vi "Process.vi"(0 "WaveformAddressSpace in":refnum<class "WaveformAddressSpace.lvclass">, 5 "Data":sgl[](array[numeric])=[0.0, 0.0, 0.0, 0.0], 9 "Iteration":i32, 11 "error in (no error)":errorcluster, 12 "FirstIteration":bool) -> (4 "WaveformAddressSpace out":refnum<class "WaveformAddressSpace.lvclass">, 6 "Acq Loop Ticks":u32, 10 "stop":bool, 15 "error out":errorcluster)   [LabVIEW 2017, in "WaveformAddressSpace.lvclass"]
uses:
  WaveformAddressSpace.lvclass
  WaveformAddressSpace.lvclass/WaveformAddressSpace.ctl
  <vilib>/rvi/DataTransferAndStorage/Container/Common/niFpgaContainerExecOnDevCompGetState.vi
  <vilib>/rvi/Emulation/niFpgaEmulationIsFPGAContextNoSignature.vi
  <vilib>/rvi/DataTransferAndStorage/Container/Common/niFpgaContainerGetUniqueNameForEmu.vi
  <vilib>/rvi/Memory/Memory_Emulation/niFpgaMemoryEmulationCacheClearOnFirstRun.vi
  <vilib>/rvi/Memory/Memory_Emulation/nirvimemoryEmulationManagerCache_MakeExclusive.vi
  <vilib>/rvi/Memory/Memory_Emulation/niFpgaMemoryEmulationValidateCache.vi
  <vilib>/rvi/Memory/Memory_Emulation/nirvimemoryEmulationManagerCache_InsertValue.vi
  <vilib>/Utility/error.llb/Clear Errors.vi
  <vilib>/rvi/Memory/Memory_Emulation/nirvimemoryEmulationManagerCache_ReleaseExclusive.vi
  <vilib>/rvi/Memory/Memory_Emulation/nirvimemoryEmulationManagerCache_GetValue.vi
  <vilib>/rvi/Memory/Memory_Emulation/nirvimemoryEmulationManagerCache_SetValue.vi
  <vilib>/rvi/Emulation/niFpgaProcessEmulError.vi
  <vilib>/rvi/Emulation/niFpgaSctlEmulationGetInTimedLoop.vi
  <vilib>/rvi/errors/niFpgaSetErrorForExecOnDevCompSimple.vi
  <vilib>/rvi/eio/common/nirviEmuReportErrorAndStop.vi
  <vilib>/rvi/FIFO/Fifo_Resource/nirvififoEmulationSetSize.vi
  <vilib>/rvi/FIFO/Fifo_Resource/nirviFifoEmulationQueueMgr.vi
  <instcachedir>/0/nirviFifoEmulationQueueMgr_E5CAEC123FF24DC58D834DCA3CDAA9B5.lvgen/nirviFifoEmulationQueueMgr_E5CAEC123FF24DC58D834DCA3CDAA9B5_002.vi
  <vilib>/rvi/FIFO/Fifo_Resource/nirvififoEmulationDetermineInputValidOut.vi
  <vilib>/rvi/FIFO/Fifo_Resource/nirvififoEmulationCreateLock.vi
  <vilib>/rvi/FIFO/Fifo_Resource/nirvififoEmulationObtainLock.vi
  <vilib>/rvi/FIFO/Fifo_Resource/nirvififoEmulationReleaseLock.vi
  <vilib>/rvi/occurrence/nirviWaitOnOccurrenceBase.vi
  <vilib>/rvi/errors/nirviReportUnexpectedCaseInternalError.vi
  <vilib>/rvi/errors/nirviReportUnexpectedCaseInternalError (U32).vi
  <vilib>/rvi/interface/RandomDataEmulation/niFpgaRandomDataHandleErrors.vi
  <vilib>/rvi/DataTransferAndStorage/Container/XNode/niFpgaContainer.xnode
  <vilib>/rvi/DataTransferAndStorage/Register/Emulation/niFpgaRegisterEmulationRefIn.vi
  <vilib>/rvi/FIFO/Fifo_Resource/niFpgaFifoEmulationRefIn.vi
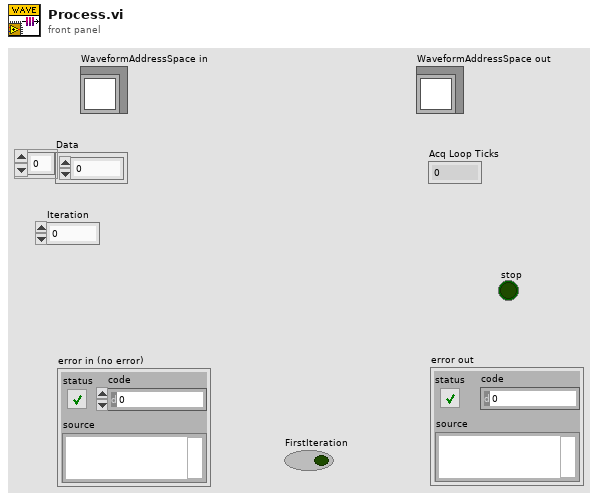
[diagram p1: front panel]
types:
  T1 = typedef "WaveformAddressSpace.lvclass/Registers.ctl" = cluster{"oclk_freq":refnum<k21>, "data_rate":refnum<k21>, "oclk_div":refnum<k21>, "oclk_mult":refnum<k21>, "AcquisitionType":refnum<k21>, "SamplesPerChan":refnum<k21>, "NumberOfChannels":refnum<k21>, "stop":refnum<k21>, "FIFO":refnum<k21>, "FirstRead":refnum<k21>, "ErrorCode":refnum<k21>, "ChannelCount":refnum<k21>, "Finished":refnum<k21>, "DMA_FIFO_Full":refnum<k21>, "ModuleUnderflow":refnum<k21>, "ConfigReadyIRQ":refnum<k21>, "ConfigReadyAck":refnum<k21>, "SynchStartIRQ":refnum<k21>, "SynchStartAck":refnum<k21>, "UnderflowCount":refnum<k21>, "FirstReadReset":refnum<k21>}
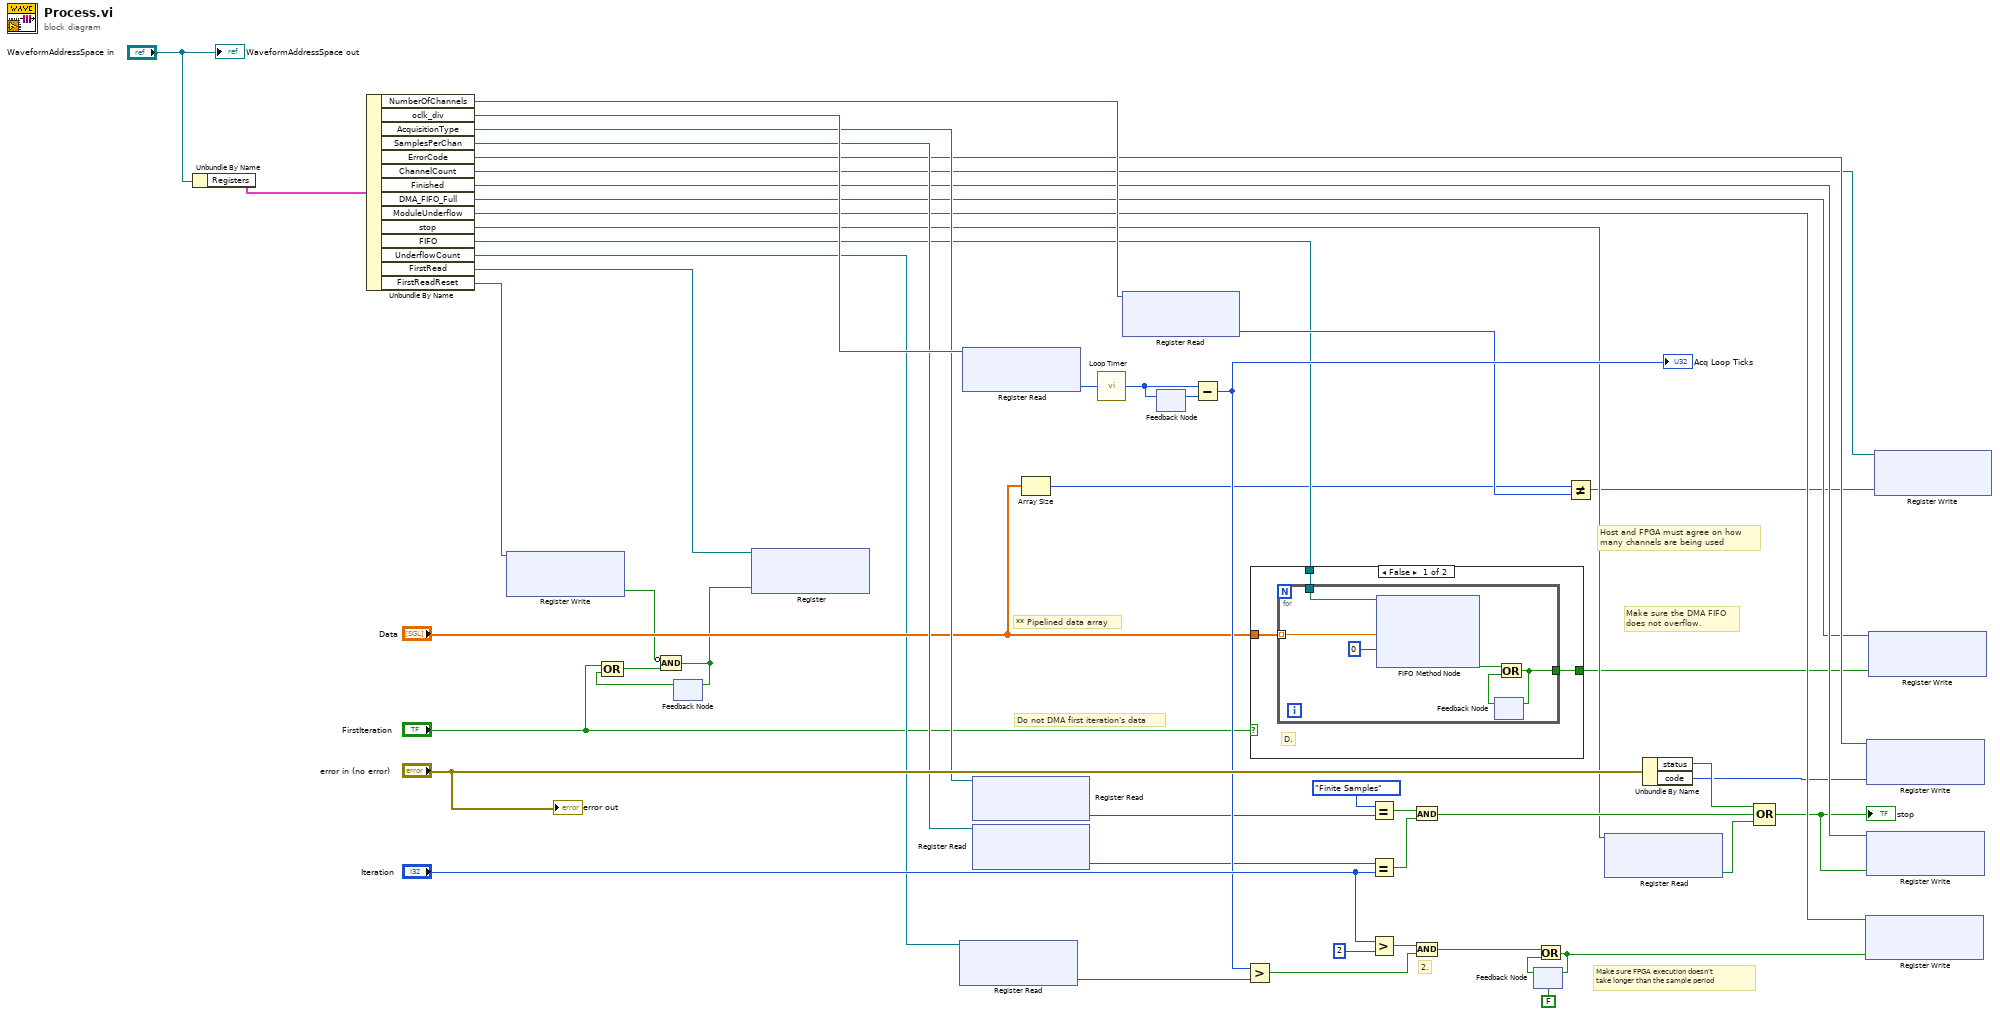
[diagram p0: block diagram]
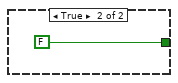
[diagram p2: hidden frame]
diagram:
  # "** Pipelined data array"
  # "2."
  # "Do not DMA first iteration's data"
  # "Host and FPGA must agree on how \nmany channels are being used"
  # "Make sure the DMA FIFO\ndoes not overflow."
  # "Make sure FPGA execution doesn't\ntake longer than the sample period"
  n1 = Unbundle By Name("WaveformAddressSpace in") -> ("Registers"=w8:T1)
  n2 = Unbundle By Name(w8) -> ("NumberOfChannels"=w33:refnum<k21>, "oclk_div"=w31:refnum<k21>, "AcquisitionType"=w29:refnum<k21>, "SamplesPerChan"=w27:refnum<k21>, "ErrorCode"=w25:refnum<k21>, "ChannelCount"=w24:refnum<k21>, "Finished"=w23:refnum<k21>, "DMA_FIFO_Full"=w22:refnum<k21>, "ModuleUnderflow"=w21:refnum<k21>, "stop"=w20:refnum<k21>, "FIFO"=w19:refnum<k21>, "UnderflowCount"=w11:refnum<k21>, "FirstRead"=w7:refnum<k21>, "FirstReadReset"=w6:refnum<k21>)
  n3 = xnode "Register Write"("Register In"=w6) -> ("Data"=w5:bool)  [unwired: 1 out]
  n4 = feedback #1() -> (w2:bool)  [unwired: 1 in]
  n5 = Compound Arithmetic op=OR("FirstIteration", w2) -> (w3:bool)
  n6 = Compound Arithmetic op=AND(invert w5, w3) -> (w4:bool)
  n7 = feedback-in #1(w4) -> ()
  n8 = xnode "Register"("Data"=w4, "Register In"=w7) -> ()  [unwired: 1 out]
  n9 = xnode ("Register Read")("Register In"=w11) -> ("Data"=w10:u32)  [unwired: 1 out]
  n10 = xnode ("Register Read")("Register In"=w31) -> ("Data"=w30:u32)  [unwired: 1 out]
  n11 = xnode ("Register Read")("Register In"=w29) -> ("Data"=w28:u16)  [unwired: 1 out]
  n12 = xnode ("Register Read")("Register In"=w27) -> ("Data"=w26:i32)  [unwired: 1 out]
  n13 = Array Size(array="Data") -> (size(s)=w12:i32)
  n14 = call "Loop Timer"("Count(Ticks)"=w30) -> ("Tick Count(Ticks)"=w34:u32)
  n15 = xnode ("Register Read")("Register In"=w33) -> ("Data"=w32:i32)  [unwired: 1 out]
  n16 = feedback #2() -> (w35:u32)  [unwired: 1 out]
  n17 = feedback-in #2(w34) -> ()
  n18 = Subtract(x=w34, y=w35) -> (x-y=w41:u32)
  "Acq Loop Ticks" <- w41
  n19 = Greater?(x=w41, y=w10) -> (0:w38:bool)
  n20 = case shown="False" "FirstIteration" {
    tunnel: [w53 FALSE] -> w17
    tunnel: "Data" -> [w52 _]
    tunnel: w19 -> [w51 _]
    frame False {
      # "D."
      n21 = for {
        tunnel: [w58] -> w53
        tunnel: w52 -> [w55] mode=indexing
        tunnel: w51 -> [w54]
        n22 = xnode ("FIFO Method Node")("Element"=w55, "Timeout"=0, "FIFO In"=w54) -> ("Timed Out?"=w56:bool)  [unwired: 1 out]
        n23 = feedback #3() -> (w59:bool)  [unwired: 1 in]
        n24 = Or(x=w56, y=w59) -> (x .or. y?=w58:bool)
        n25 = feedback-in #3(w58) -> ()
      }
    }
    frame True {
    }
  }
  n26 = Equal?(x=enum16{"Finite Samples", "Continuous Samples"}."Finite Samples" ("y"), y=w28) -> (x = y?=w47:bool)
  n27 = Equal?(x=w26, y="Iteration") -> (x = y?=w48:bool)
  n28 = Greater?(x="Iteration", y=2) -> (0:w39:bool)
  n29 = And(x=w47, y=w48) -> (x .and. y?=w49:bool)
  n30 = And(x=w39, y=w38) -> (x .and. y?=w46:bool)
  n31 = feedback #4(FALSE) -> (w44:bool)
  n32 = Or(x=w46, y=w44) -> (x .or. y?=w15:bool)
  n33 = feedback-in #4(w15) -> ()
  n34 = Not Equal?(x=w12, y=w32) -> (x != y?=w18:bool)
  n35 = xnode ("Register Read")("Register In"=w20) -> ("Data"=w36:bool)  [unwired: 1 out]
  n36 = Unbundle By Name("error in (no error)") -> ("status"=w43:bool, "code"=w14:i32)
  n37 = Compound Arithmetic op=OR(w43, w49, w36) -> (w16:bool)
  "stop" <- w16
  n38 = xnode ("Register Write")("Data"=w15, "Register In"=w21) -> ()  [unwired: 1 out]
  n39 = xnode ("Register Write")("Data"=w14, "Register In"=w25) -> ()  [unwired: 1 out]
  n40 = xnode ("Register Write")("Data"=w16, "Register In"=w23) -> ()  [unwired: 1 out]
  n41 = xnode ("Register Write")("Data"=w17, "Register In"=w22) -> ()  [unwired: 1 out]
  n42 = xnode ("Register Write")("Data"=w18, "Register In"=w24) -> ()  [unwired: 1 out]
  "WaveformAddressSpace out" <- "WaveformAddressSpace in"
  "error out" <- "error in (no error)"
